vi "Set Acquisition Mode.vi"(8 "error in (no error)":errorcluster, 10 "nMode":T1, 11 "nSensorIP":u32) -> (0 "error out":errorcluster, 3 "function return":i32)   [LabVIEW 2022 SP3, in "BonTechDetector.lvlib"]
doc: "extern \"C\" BONTECHLIBRARY_API int __stdcall SetAcquisitionMode(unsigned int nSensorIP, int nMode);"
uses:
  BonTechDetector.lvlib
  Controls/Acquisition Modes.ctl
  C:/Users/Sandeep/Downloads/The Oracle-lv2021/Image Acquisition/Child Classes/BonTechFlatPanel/BonTechWrapperLibrary.dll
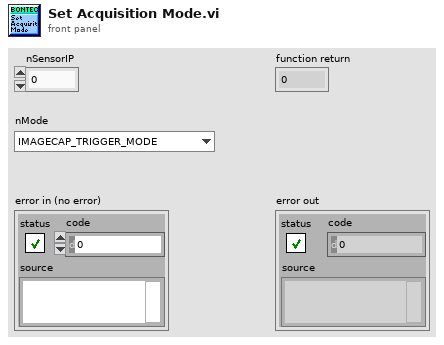
[diagram p1: front panel]
types:
  T1 = typedef "BonTechDetector.lvlib/Acquisition Modes.ctl" = enum32{"IMAGECAP_TRIGGER_MODE", "IMAGECAP_AED_MODE", "IMAGECAP_SOFTTRIGGER_MODE", "IMAGECAP_AVG_COUNT_MODE", "IMAGECAP_AVG_AED_MODE", "IMAGECAP_CONTINUOUS_MODE", "IMAGECAP_VIEWER_MODE", "IMAGECAP_CONTINUOUS_BINNING_MODE"}
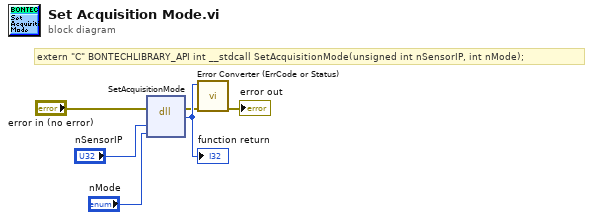
[diagram p0: block diagram]
diagram:
  # "extern \"C\" BONTECHLIBRARY_API int __stdcall SetAcquisitionMode(unsigned int nSensorIP, int nMode);"
  n1 = dll-call lib="C:/Users/Sandeep/Downloads/The Oracle-lv2021/Image Acquisition/Child Classes/BonTechFlatPanel/BonTechWrapperLibrary.*" fn="SetAcquisitionMode"(error in="error in (no error)", "nSensorIP"="nSensorIP", "nMode"="nMode") -> (error out=w2:errorcluster, "return type"=w6:i32)  [unwired: 4 in, 1 out]
  "function return" <- w6
  n2 = call "Error Converter (ErrCode or Status).vi"("error in (no error)"=w2, "error code"=w6) -> ("error out"=→"error out":errorcluster)  [unwired: 9 in]
